vi "EPICS_Client_PVs_Builder_20160201.vi"(8 "error in (no error)":errorcluster, 10 "PV_names":string[](array[string]), 11 "EPICS Server URL in":string="\\\\.\\Client Library\\EPICS Client_print") -> (0 "error out":errorcluster, 3 "EPICS Client ref out":refnum<data-value>)   [LabVIEW 2013]
uses:
  <vilib>/variable/tagger/epics/API/internal/EPICSClientClass/EPICSClient.lvclass
  <vilib>/variable/tagger/epics/API/NI_EPICS_Client.lvlib
panel:
  # "psp:\\\\localhost\\Client Library\\EPICS Client_print\\"
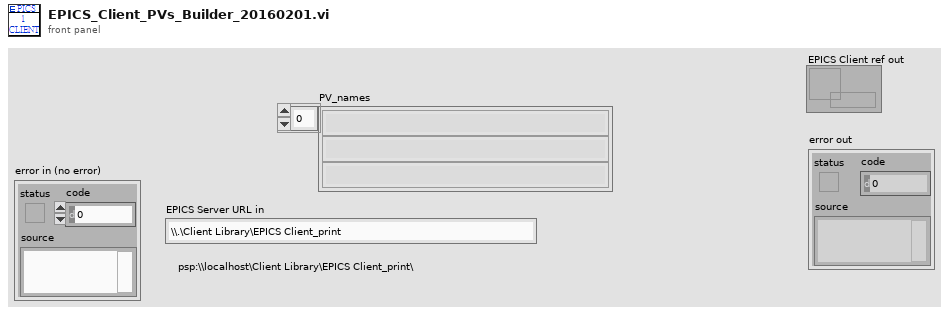
[diagram p1: front panel]
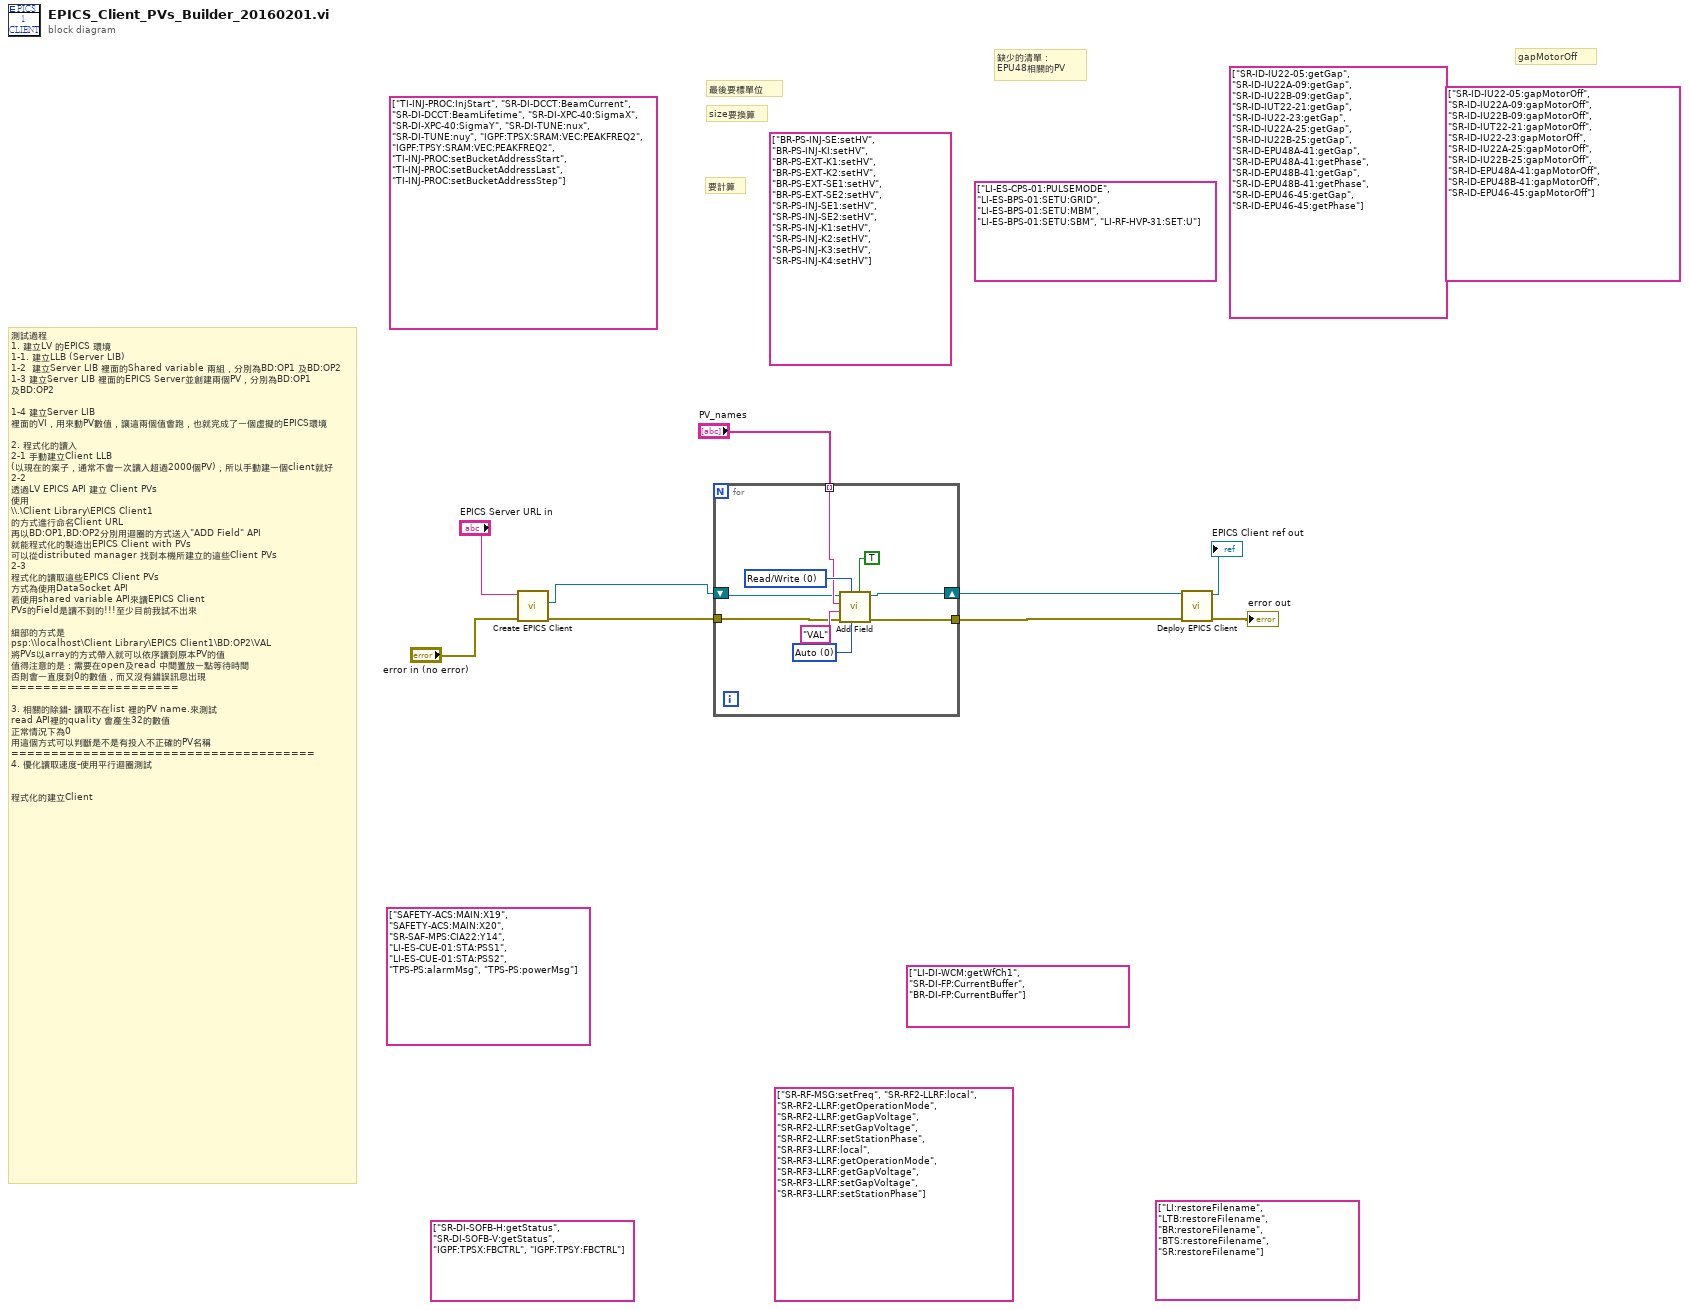
[diagram p0: block diagram]
diagram:
  (unwired) string[] ["SR-ID-IU22-05:gapMotorOff", "SR-ID-IU22A-09:gapMotorOff", "SR-ID-IU22B-09:gapMotorOff", "SR-ID-IUT22-21:gapMotorOff", "SR-ID-IU22-23:gapMotorOff", "SR-ID-IU22A-25:gapMotorOff", "SR-ID-IU22B-25:gapMotorOff", "SR-ID-EPU48A-41:gapMotorOff", "SR-ID-EPU48B-41:gapMotorOff", "SR-ID-EPU46-45:gapMotorOff"]
  (unwired) string[] ["SR-ID-IU22-05:getGap", "SR-ID-IU22A-09:getGap", "SR-ID-IU22B-09:getGap", "SR-ID-IUT22-21:getGap", "SR-ID-IU22-23:getGap", "SR-ID-IU22A-25:getGap", "SR-ID-IU22B-25:getGap", "SR-ID-EPU48A-41:getGap", "SR-ID-EPU48A-41:getPhase", "SR-ID-EPU48B-41:getGap", "SR-ID-EPU48B-41:getPhase", "SR-ID-EPU46-45:getGap", "SR-ID-EPU46-45:getPhase"]
  (unwired) string[] ["LI-ES-CPS-01:PULSEMODE", "LI-ES-BPS-01:SETU:GRID", "LI-ES-BPS-01:SETU:MBM", "LI-ES-BPS-01:SETU:SBM", "LI-RF-HVP-31:SET:U"]
  (unwired) string[] ["BR-PS-INJ-SE:setHV", "BR-PS-INJ-KI:setHV", "BR-PS-EXT-K1:setHV", "BR-PS-EXT-K2:setHV", "BR-PS-EXT-SE1:setHV", "BR-PS-EXT-SE2:setHV", "SR-PS-INJ-SE1:setHV", "SR-PS-INJ-SE2:setHV", "SR-PS-INJ-K1:setHV", "SR-PS-INJ-K2:setHV", "SR-PS-INJ-K3:setHV", "SR-PS-INJ-K4:setHV"]
  (unwired) string[] ["TI-INJ-PROC:InjStart", "SR-DI-DCCT:BeamCurrent", "SR-DI-DCCT:BeamLifetime", "SR-DI-XPC-40:SigmaX", "SR-DI-XPC-40:SigmaY", "SR-DI-TUNE:nux", "SR-DI-TUNE:nuy", "IGPF:TPSX:SRAM:VEC:PEAKFREQ2", "IGPF:TPSY:SRAM:VEC:PEAKFREQ2", "TI-INJ-PROC:setBucketAddressStart", "TI-INJ-PROC:setBucketAddressLast", "TI-INJ-PROC:setBucketAddressStep"]
  (unwired) string[] ["LI:restoreFilename", "LTB:restoreFilename", "BR:restoreFilename", "BTS:restoreFilename", "SR:restoreFilename"]
  (unwired) string[] ["SR-RF-MSG:setFreq", "SR-RF2-LLRF:local", "SR-RF2-LLRF:getOperationMode", "SR-RF2-LLRF:getGapVoltage", "SR-RF2-LLRF:setGapVoltage", "SR-RF2-LLRF:setStationPhase", "SR-RF3-LLRF:local", "SR-RF3-LLRF:getOperationMode", "SR-RF3-LLRF:getGapVoltage", "SR-RF3-LLRF:setGapVoltage", "SR-RF3-LLRF:setStationPhase"]
  (unwired) string[] ["SR-DI-SOFB-H:getStatus", "SR-DI-SOFB-V:getStatus", "IGPF:TPSX:FBCTRL", "IGPF:TPSY:FBCTRL"]
  (unwired) string[] ["LI-DI-WCM:getWfCh1", "SR-DI-FP:CurrentBuffer", "BR-DI-FP:CurrentBuffer"]
  (unwired) string[] ["SAFETY-ACS:MAIN:X19", "SAFETY-ACS:MAIN:X20", "SR-SAF-MPS:CIA22:Y14", "LI-ES-CUE-01:STA:PSS1", "LI-ES-CUE-01:STA:PSS2", "TPS-PS:alarmMsg", "TPS-PS:powerMsg"]
  # "要計算"
  # "gapMotorOff"
  # "最後要標單位"
  # "size要換算"
  # "缺少的清單：\nEPU48相關的PV"
  # "測試過程\n1. 建立LV 的EPICS 環境\n1-1. 建立LLB (Server LIB) \n1-2  建立Server LIB 裡面的Shared variable 兩組，分別為BD:OP1 及BD:OP2\n1-3 建立Server LIB 裡面的EPICS Server並創建兩個PV，分別為BD:OP1 及BD:OP2\n\n1-4 建立Server LIB 裡面的VI，用來動PV數值，讓這兩個值會跑，也就完成了一個虛擬的EPICS環境\n\n2. 程式化的讀入\n2-1 手動建立Client LLB (以現在的案子，通常不會一次讀入超過2000個PV)，所以手動建一個client就好\n2-2\n透過LV EPICS API 建立 Client PVs\n使用\n\\\\.\\Client Library\\EPICS Client1\n的方式進行命名Client URL\n再以BD:OP1,BD:OP2分別用迴圈的方式送入\"ADD Field\" API\n就能程式化的製造出EPICS Client with PVs\n可以從distributed manager 找到本機所建立的這些Client PVs\n2-3\n程式化的讀取這些EPICS Client PVs\n方式為使用DataSocket API\n若使用shared variable API來讀EPICS Client PVs的Field是讀不到的!!!至少目前我試不出來\n\n細部的方式是\npsp:\\\\localhost\\Client Library\\EPICS Client1\\BD:OP2\\VAL\n將PVs以array的方式帶入就可以依序讀到原本PV的值\n值得注意的是：需要在open及read 中間置放一點等待時間\n否則會一直度到0的數值，而又沒有錯誤訊息出現\n=====================\n\n3. 相關的除錯- 讀取不在list 裡的PV name.來測試\nread API裡的quality 會產生32的數值\n正常情況下為0\n用這個方式可以判斷是不是有投入不正確的PV名稱\n======================================\n4. 優化讀取速度-使用平行迴圈測試\n\n\n程式化的建立Client"
  n1 = call <vilib>:"Create EPICS Client.vi"("error in (no error)"="error in (no error)", "EPICS Client URL in"="EPICS Server URL in") -> ("error out"=w5:errorcluster, "EPICS Client ref"=w2:refnum<data-value>)  [unwired: 7 in, 1 out]
  n2 = for {
    tunnel: w5 -> [w15]
    tunnel: [w12] -> w4
    tunnel: "PV_names" -> [w11] mode=indexing
    shift-right: [w18] -> w8
    shift-left: w2 -> [w10]
    w16 = u16 0 items=["Auto", "Double", "Bool", "String", "Short", "Float", "Enum", "Long", "Array of Double"] ("data type")
    w13 = u16 0 items=["Read/Write", "Read Only", "Write Only"] ("access type")
    n3 = call <vilib>:"Add Field.vi"("add record? (T)"=TRUE, "data type"=w16, "access type"=w13, "error in (no error)"=w15, "field name"="VAL", "record name"=w11, "EPICS Client ref in"=w10) -> ("error out"=w12:errorcluster, "EPICS Client ref out"=w18:refnum<data-value>)  [unwired: 1 in, 2 out]
  }
  n4 = call <vilib>:"Deploy EPICS Client.vi"("error in (no error)"=w4, "EPICS Client ref in"=w8) -> ("error out"=→"error out":errorcluster, "EPICS Client ref out"=→"EPICS Client ref out":refnum<data-value>)  [unwired: 8 in]
